vi "Image_Processing_Queue_Info.vi"(11 "Data":T1={"L16 Linear Actuator"="", "XE 1000 Pump"="", "Camera1"="", "Camera2"="", "Img_Capt"=FALSE, "Actuator"=FALSE, "Pump"=FALSE, "Cam 1"=FALSE, "Cam 2"=FALSE, "Empty_Refill"=FALSE, "Crop"=FALSE, "Light intensity"=0, "Exposure Time"=0.0, "Sample Name"="", "Operator"="", "Calibration 1"=path "", "Calibration 2"=path "", "Framerate"=0, "Timeout Sample"=0, "Collection date"="", "Sample size threshold"=0, "Empty start"=0, "Command"="", "Station"="", "Species Name"="", "Other Notes"="", "Aperture"=enum."Item 0", "Image Process Queue Size"=500, "Image Save Queue Size"=500, "Overload threshold"=500, "Max Framerate"=100, "Rectangle 1"={"Left"=0, "Top"=0, "Right"=0, "Bottom"=0, "Rotation"=0.0}, "Rectangle 2"={"Left"=0, "Top"=0, "Right"=0, "Bottom"=0, "Rotation"=0.0}, "Detection Region %"=0.0, "Detect 1"=path "C:/Users/au540322/Desktop/IHS_Project/images/Debris/Debris_0/Debris_0_2019_06_01-23-32-49-686.PNG", "Detect 2"=path "C:/Users/au540322/Desktop/IHS_Project/images/Debris/Debris_0/Debris_0_2019_06_01-23-32-49-686.PNG", "Max large object threshold"=0, "Open(T)/Close(F)"=FALSE, "Img_Capt Begin"=FALSE, "Dispense Speed"=100, "Flush Size"=100, "Location"="Station", "Latitude"="Station", "Longitude"="Station", "Determiner"="Station", "Sex"="Station", "Camera1_Img"=refnum, "Camera2_Img"=refnum, "Img1_Orig_Disp"=refnum, "Img2_Orig_Disp"=refnum, "Img1_Orig_RGB"=refnum, "Img2_Orig_RGB"=refnum, "Blue_Plane_Extract"=refnum, "Subtracted_Plane"=refnum, "Img1_Binary"=refnum, "Img2_Binary"=refnum, "Crop_Mask"=refnum, "Img1_Save"=refnum, "Img2_Save"=refnum, "Img1_Cali_Full"=refnum, "Img2_Cali_Full"=refnum, "Img1_Cali_Detect"=refnum, "Img2_Cali_Detect"=refnum, "Cam 1 queue"=refnum, "Cam 2 queue"=refnum, "Cam 1 - save queue"=refnum, "Cam 2 - save queue"=refnum, "Overlay_Ring"=0, "SystemVersion"=0, "System Serial"="", "Legacy Cam Attributes"=FALSE} {"SystemVersion" items=["Standard", "XL"]; "Overlay_Ring" items=["Session Data", "Extended Setup", "Buffer", "Camera", "Dispenser", "Stats", "Connections"]; "Flush Size" min=1; "Dispense Speed" min=1; "Rectangle 2"."Rotation" format="%.2f"; "Rectangle 2"."Left" scale=0.0..1024.0; "Rectangle 2"."Right" scale=0.0..1024.0; "Rectangle 1"."Rotation" format="%.2f"; "Rectangle 1"."Left" scale=0.0..1024.0; "Rectangle 1"."Right" scale=0.0..1024.0; "Max Framerate" min=1; "Overload threshold" min=1; "Image Save Queue Size" min=1; "Image Process Queue Size" min=1; "Empty start" min=1; "Sample size threshold" min=1; "Framerate" min=1; "Light intensity" scale=0.0..100.0}) -> (0 "Max Queue Size":i32, 1 "Queue data":T5, 3 "Last Image?":bool)   [LabVIEW 2022 SP3]
uses:
  controls/Data.ctl
  <vilib>/userdefined/High Color/IMAQdx.ctl
  <vilib>/vision/Image Controls.llb/IMAQ Image.ctl
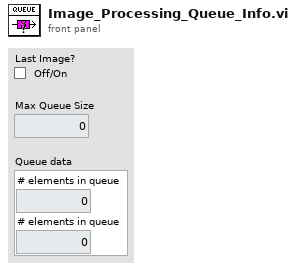
[diagram p1: front panel]
types:
  T1 = typedef "Data.ctl" = cluster{"L16 Linear Actuator":refnum<visa-resource-name>, "XE 1000 Pump":refnum<visa-resource-name>, "Camera1":T2, "Camera2":T2, "Img_Capt":bool, "Actuator":bool, "Pump":bool, "Cam 1":bool, "Cam 2":bool, "Empty_Refill":bool, "Crop":bool, "Light intensity":i32, "Exposure Time":dbl, "Sample Name":string, "Operator":string, "Calibration 1":path, "Calibration 2":path, "Framerate":i32, "Timeout Sample":i32, "Collection date":string, "Sample size threshold":i32, "Empty start":u32, "Command":string, "Station":string, "Species Name":string, "Other Notes":string, "Aperture":enum32{"Item 0", "Item 1", "Item 2", "Item 3"}, "Image Process Queue Size":i32, "Image Save Queue Size":i32, "Overload threshold":i32, "Max Framerate":i32, "Rectangle 1":T3, "Rectangle 2":T3, "Detection Region %":dbl, "Detect 1":path, "Detect 2":path, "Max large object threshold":i32, "Open(T)/Close(F)":bool, "Img_Capt Begin":bool, "Dispense Speed":i32, "Flush Size":i32, "Location":string, "Latitude":string, "Longitude":string, "Determiner":string, "Sex":string, "Camera1_Img":T4, "Camera2_Img":T4, "Img1_Orig_Disp":T4, "Img2_Orig_Disp":T4, "Img1_Orig_RGB":T4, "Img2_Orig_RGB":T4, "Blue_Plane_Extract":T4, "Subtracted_Plane":T4, "Img1_Binary":T4, "Img2_Binary":T4, "Crop_Mask":T4, "Img1_Save":T4, "Img2_Save":T4, "Img1_Cali_Full":T4, "Img2_Cali_Full":T4, "Img1_Cali_Detect":T4, "Img2_Cali_Detect":T4, "Cam 1 queue":refnum<queue>, "Cam 2 queue":refnum<queue>, "Cam 1 - save queue":refnum<queue>, "Cam 2 - save queue":refnum<queue>, "Overlay_Ring":u16, "SystemVersion":u16, "System Serial":string, "Legacy Cam Attributes":bool}
  T2 = typedef "IMAQdx.ctl" = refnum<k21>
  T3 = typedef "IMAQ Rectangle" = cluster{"Left":i32, "Top":i32, "Right":i32, "Bottom":i32, "Rotation":dbl}
  T4 = typedef "IMAQ Image.ctl" = refnum<image>
  T5 = cluster{"# elements in queue":i32, "# elements in queue":i32}
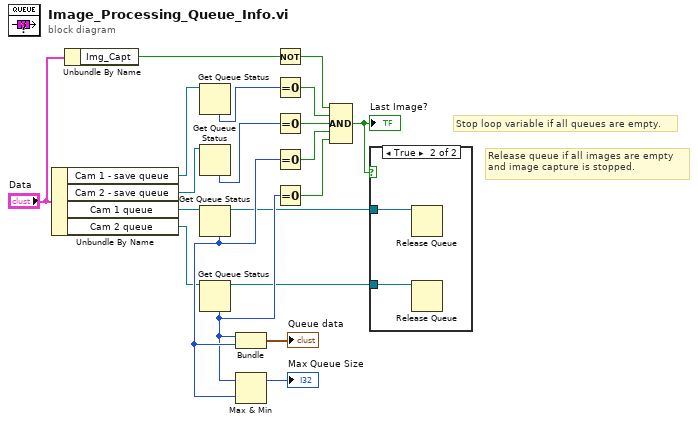
[diagram p0: block diagram]
diagram:
  # "Stop loop variable if all queues are empty."
  # "Release queue if all images are empty \nand image capture is stopped."
  n1 = Unbundle By Name("Data") -> ("Cam 1 - save queue"=w2:refnum<queue>, "Cam 2 - save queue"=w5:refnum<queue>, "Cam 1 queue"=w9:refnum<queue>, "Cam 2 queue"=w10:refnum<queue>)
  n2 = Unbundle By Name("Data") -> ("Img_Capt"=w1:bool)
  n3 = Get Queue Status(queue=w2) -> (# elements in queue=w3:i32)  [unwired: 2 in, 7 out]
  n4 = Get Queue Status(queue=w5) -> (# elements in queue=w4:i32)  [unwired: 2 in, 7 out]
  n5 = Get Queue Status(queue=w9) -> (queue out=w6:refnum<queue>, # elements in queue=w19:i32)  [unwired: 2 in, 6 out]
  n6 = Get Queue Status(queue=w10) -> (queue out=w7:refnum<queue>, # elements in queue=w18:i32)  [unwired: 2 in, 6 out]
  n7 = Bundle("# elements in queue"=w18, "# elements in queue"=w19) -> (→"Queue data":T5)  [unwired: 1 in]
  n8 = Max & Min(x=w18, y=w19) -> (max(x,y)=→"Max Queue Size":i32)  [unwired: 1 out]
  n9 = Not(x=w1) -> (.not. x?=w15:bool)
  n10 = Equal To 0?(x=w3) -> (x = 0?=w14:bool)
  n11 = Equal To 0?(x=w4) -> (x = 0?=w13:bool)
  n12 = Equal To 0?(x=w19) -> (x = 0?=w12:bool)
  n13 = Equal To 0?(x=w18) -> (x = 0?=w11:bool)
  n14 = Compound Arithmetic op=AND(w15, w14, w13, w12, w11) -> (w8:bool)
  "Last Image?" <- w8
  n15 = case shown="True" w8 {
    tunnel: w7 -> [_ w22]
    tunnel: w6 -> [_ w21]
    frame False {
    }
    frame True {
      n16 = Release Queue(queue=w21) -> ()  [unwired: 2 in, 3 out]
      n17 = Release Queue(queue=w22) -> ()  [unwired: 2 in, 3 out]
    }
  }
